vi "deleteDeviceLow.vi"(8 "error in (no error)":errorcluster, 9 "S/N IN":string, 10 "Device Type In":T1=enum."k4b2", 11 "reference in":refnum<class "Project Panels.lvclass">=refnum) -> (0 "error out":errorcluster={"status"=TRUE, "code"=1556, "source"="In Place Element Structure in File Controller.lvclass:getExcelFileRefs.vi->Devices Controller.lvclass:newDevice.vi->Project Panels.lvclass:newItem.vi->Project Panels.lvclass:products.vi->GUI Controller.lvclass:operate.vi->Master Controller.lvclass:operate.vi->main.vi"}, 2 "saved?":bool, 3 "reference out":refnum<class "Project Panels.lvclass">)   [LabVIEW 2016, in "Project Panels.lvclass"]
uses:
  Project Panels.lvclass
  SYS/Devices Controller_llb/deviceType.ctl
  deviceState.ctl
  SYS/Devices Controller_llb/Devices Controller.lvclass
panel:
  out "title":string="Deleting ...."
  out "O2 Exp Date (mm-aa)":string
  out "Serviced by":string
  out "O2 Last Changed (mm-aa)":string
  out "Follow Up Accepeted":string
  out "Follow Up Sent":string
  out "Device Type":T1=enum."k4b2"
  out "City":string
  out "End User Email":string
  out "End User":string
  out "System's Location":string
  out "Account":string
  out "Description":string
  out "SW Version":string
  out "S/N":string
  out "statusBar":string
  in  "Delete Item":bool
  in  "Stop Button":bool
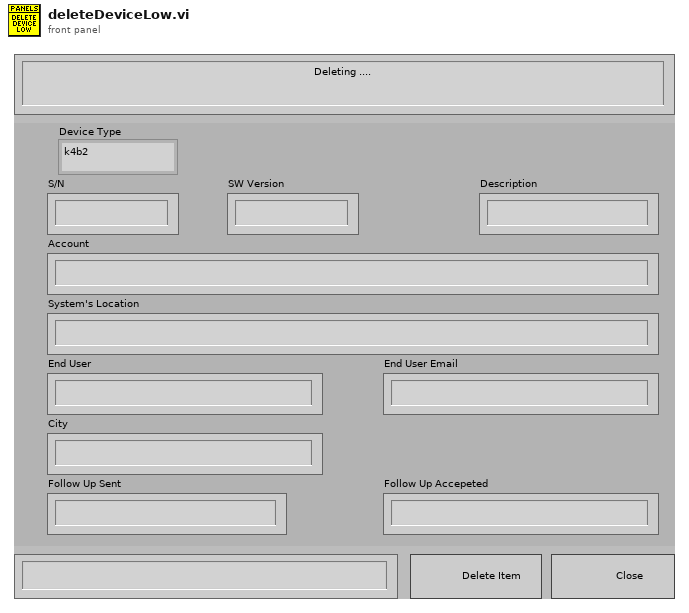
[diagram p1: front panel]
types:
  T1 = typedef "Devices Controller.lvclass/deviceType.ctl" = enum16{"k5", "k4b2", "fitmate", "cpet", "rmr", "bodyBoxPft", "bp", "pp"}
  T2 = cluster{"deviceType":T1, "S/N":string, "SW":string, "Description":string, "Account":string, "System's Location":string, "End User":string, "Email":string, "City":string, "LastChange":string, "Service By":string, "Exp Date":string, "FollowUp Sent":string, "FollowUp Accepted":string}
  T3 = typedef "Project Panels.lvclass/deviceState.ctl" = enum16{"check", "initiate", "waitEvent", "dataFromPDF", "getDetails", "TSR", "save", "close", "stop"}
  T4 = typedef "Project Panels.lvclass/ObjectAttributesRef.ctl" = refnum<data-value>
  T5 = typedef "Project Panels.lvclass/ObjectAttributes.ctl" = cluster{"MyAttribute":dbl, "device_controller_ref":refnum<class "Devices Controller.lvclass">, "file_controller_ref":refnum<class "File Controller.lvclass">, "item_controller_ref":refnum<class "Items Controller.lvclass">, "item_tables":cluster{"checkIN":string[][], "checkOUT":string[][], "storage":string[][]}, "quickbook_table":cluster{"notes":string[][]}, "notification_controller_ref":refnum<class "Notification Controller.lvclass">, "partstracking_controller_ref":refnum<class "PartsTracking Controller.lvclass">, "product_tables":cluster{"k4b2":string[][], "fitmate":string[][], "RMR":string[][], "CPET":string[][], "BP":string[][], "PP":string[][], "k5":string[][], "bb-pft":string[][]}, "rowsColour":u32[], "low_resolution?":bool, "run_python?":bool}
  T6 = cluster{"deviceType":T1, "S/N":string, "SW":string, "Description":string, "Account":string, "System's Location":string, "End User":string, "Email":string, "City":string, "LastChange":string, "Service By":string, "Exp Date":string, "FollowUp Sent":string, "FollowUp Accepted":string, "Note":string}
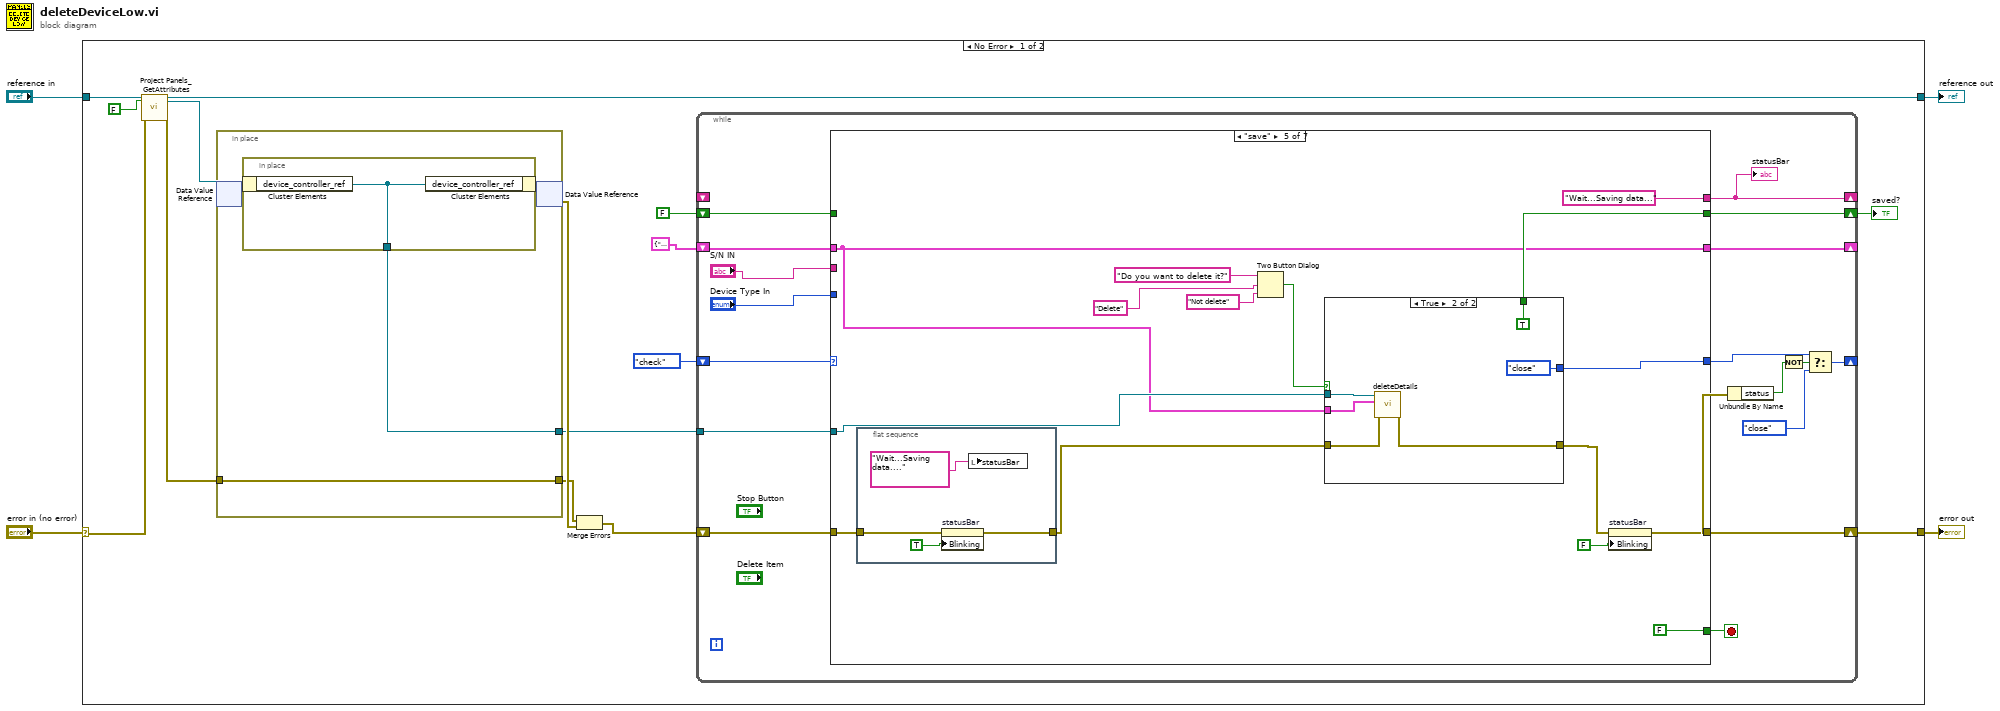
[diagram p0: block diagram]
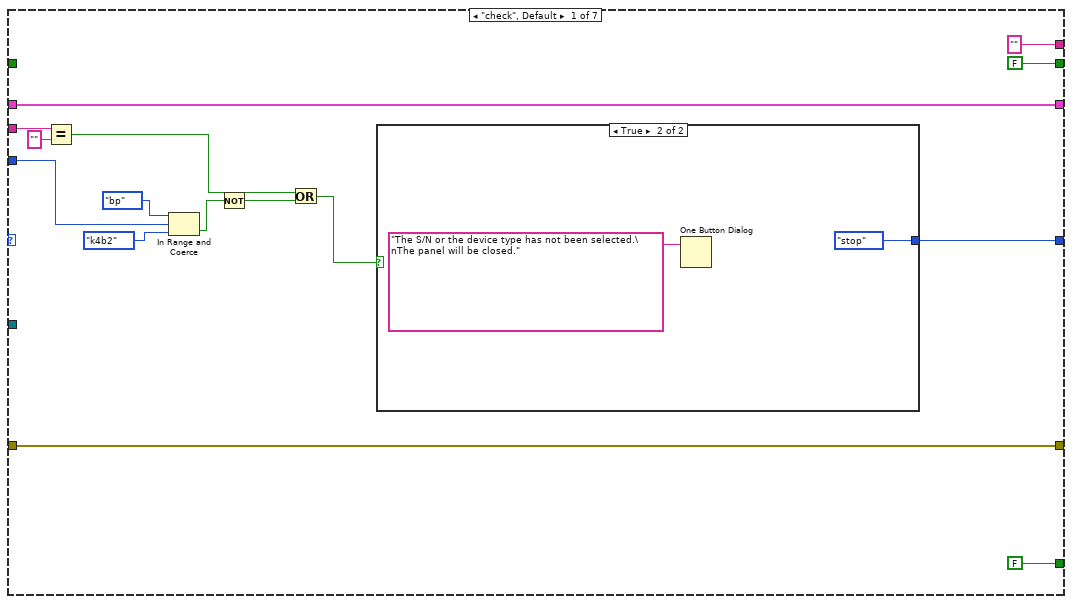
[diagram p2: hidden frame]
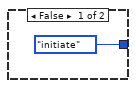
[diagram p3: hidden frame]
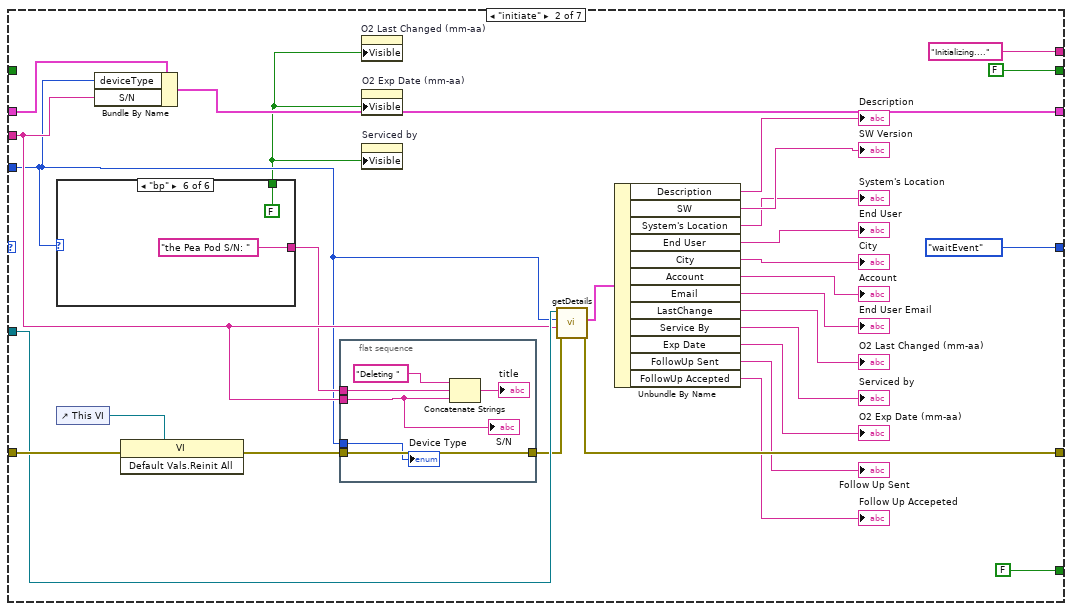
[diagram p4: hidden frame]
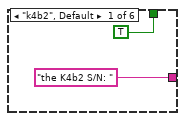
[diagram p5: hidden frame]
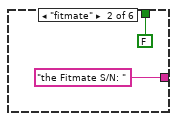
[diagram p6: hidden frame]
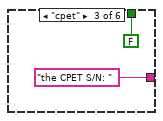
[diagram p7: hidden frame]
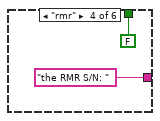
[diagram p8: hidden frame]
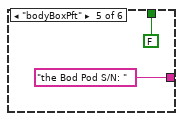
[diagram p9: hidden frame]
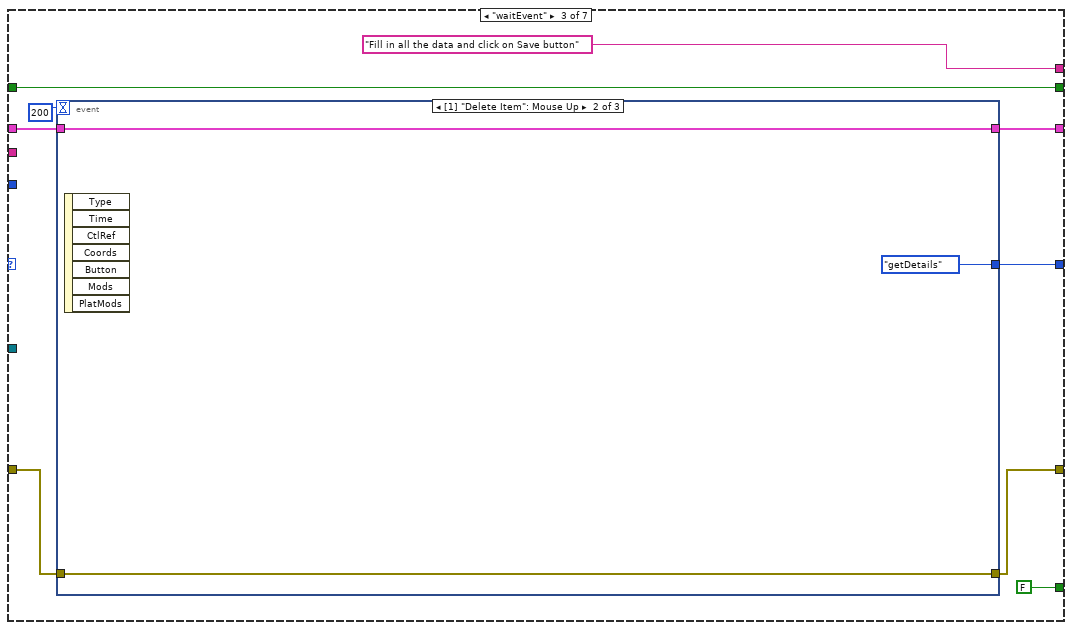
[diagram p10: hidden frame]
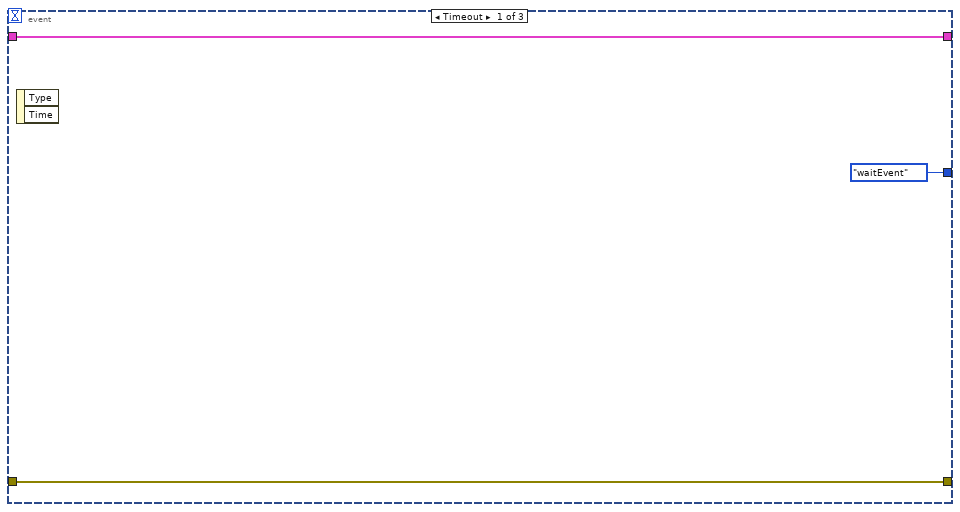
[diagram p11: hidden frame]
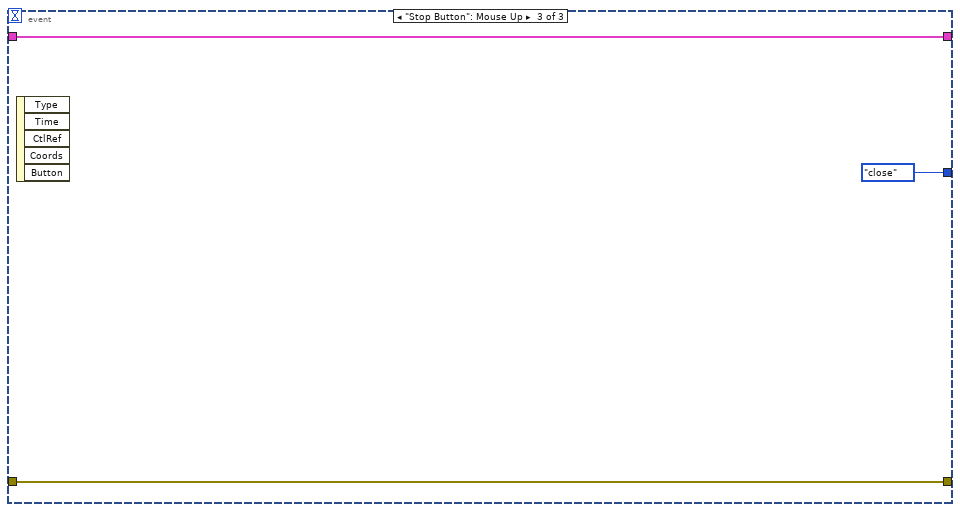
[diagram p12: hidden frame]
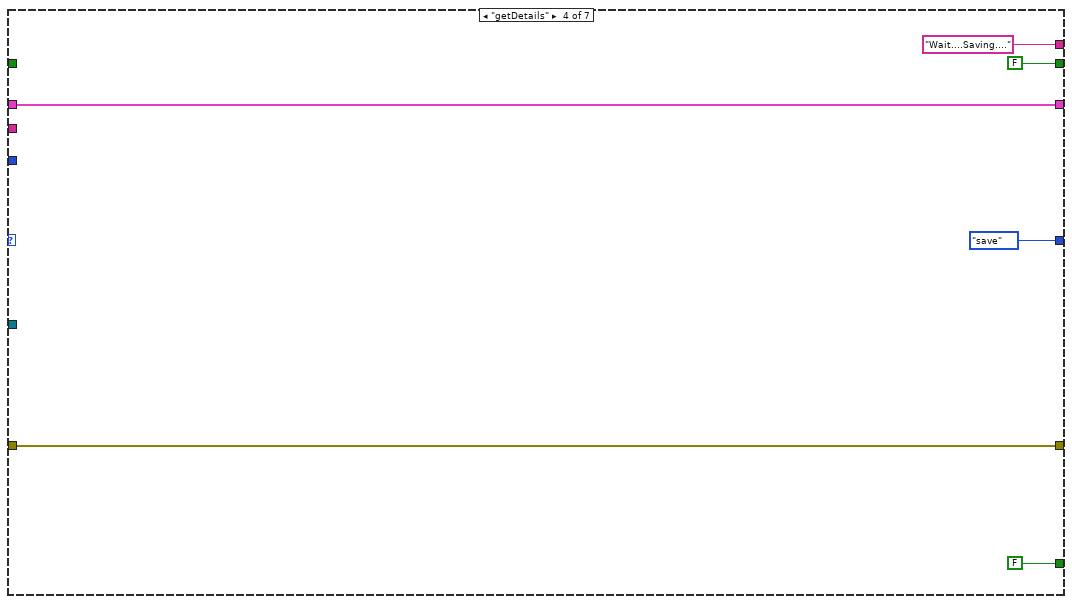
[diagram p13: hidden frame]
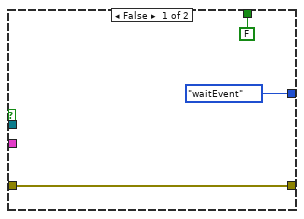
[diagram p14: hidden frame]
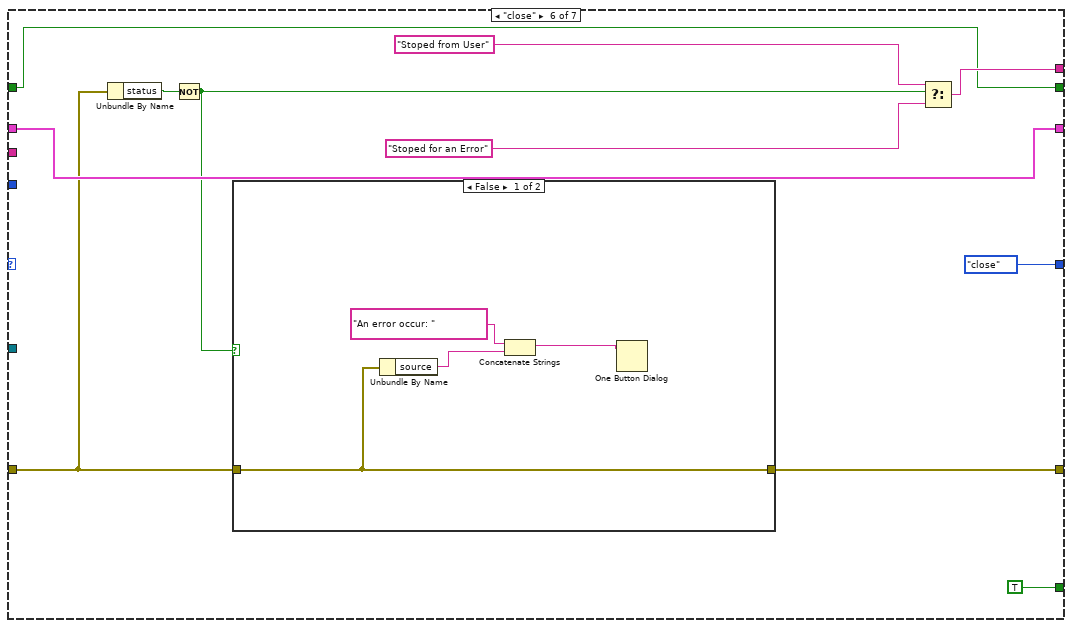
[diagram p15: hidden frame]
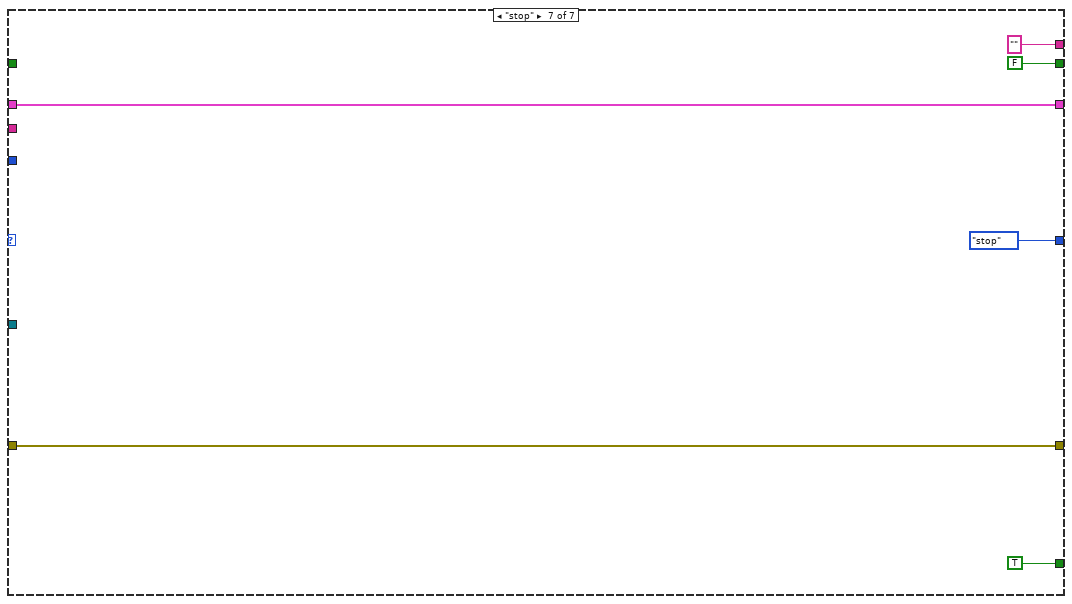
[diagram p17: hidden frame]
diagram:
  n1 = case shown="No Error" "error in (no error)" {
    selector: "error in (no error)" -> [w15 w182]
    tunnel: [w10 w182] -> w3
    tunnel: [w13 w181] -> w1
    tunnel: "reference in" -> [w17 w181]
    frame No Error {
      n2 = call "Project Panels_GetAttributes.vi"("reference in"=w17, "return data? (T)"=FALSE, "error in (no error)"=w15) -> ("reference out"=w13:refnum<class "Project Panels.lvclass">, "attributes ref"=w12:T4, "error out"=w14:errorcluster)  [unwired: 13 in, 1 out]
      n3 = in-place {
        in-place-border: w14 -> [w177]
        in-place-border: [w177] -> w18
        in-place-border: [w176] -> w8
        n4 = in-place-dvr #1(w12) -> (w178:T5)  [unwired: 1 out]
        n5 = in-place {
          in-place-border: [w180] -> w176
          n6 = in-place-cluster #2(w178) -> ("device_controller_ref"=w180:refnum<class "Devices Controller.lvclass">)
          n7 = in-place-cluster #2("device_controller_ref"=w180) -> (w179:T5)
        }
        n8 = in-place-dvr #1(w179) -> (w19:errorcluster)  [unwired: 1 out]
      }
      n9 = Merge Errors(w18, w19) -> (w11:errorcluster)
      n10 = while {
        shift-right: [w25] -> w10
        shift-left: w11 -> [w36]
        shift-right: [w26] -> _
        shift-left: deviceState."check" ("state") -> [w35]
        shift-right: [w33] -> _
        shift-left: T2 {"deviceType"=enum."k5", "S/N"="", "SW"="", "Description"="", "Account"="", "System's Location"="", "End User"="", "Email"="", "City"="", "LastChange"="", "Service By"="", "Exp Date"="", "FollowUp Sent"="", "FollowUp Accepted"=""} ("details") -> [w32]
        shift-right: [w31] -> _
        shift-left: _ -> [_]
        tunnel: w8 -> [w30]
        shift-right: [w29] -> w5
        shift-left: FALSE -> [w28]
        stop <- w34 stop-if-true
        n11 = case shown="\"save\"" w35 {
          tunnel: w36 -> [w51 w78 w105 w125 w135 w159 w174]
          tunnel: [w51 w77 w104 w125 w132 w158 w174] -> w25
          tunnel: [FALSE FALSE FALSE FALSE FALSE TRUE TRUE] -> w34
          tunnel: [w38 deviceState."waitEvent" ("state") w109 deviceState."save" ("f") w139 deviceState."close" ("f") deviceState."stop" ("f")] -> w27
          tunnel: "Device Type In" -> [w47 w68 _ _ _ _ _]
          tunnel: [w48 w73 w102 w120 w136 w161 w172] -> w33
          tunnel: w32 -> [w48 w74 w103 w120 w136 w161 w172]
          tunnel: ["" ("title") "Initializing...." ("statusBar") "Fill in all the data and click on Save button" ("statusBar") "Wait....Saving...." ("title") "Wait...Saving data..." ("title") w160 "" ("title")] -> w31
          tunnel: w30 -> [_ w76 _ _ w138 _ _]
          tunnel: [FALSE FALSE w106 FALSE w137 w156 FALSE] -> w29
          tunnel: w28 -> [_ _ w106 _ _ w156 _]
          tunnel: "S/N IN" -> [w44 w72 _ _ _ _ _]
          frame "check", Default {
            n12 = Equal?(x=w44, y="") -> (x = y?=w41:bool)
            n13 = In Range and Coerce(upper limit=deviceType."bp", x=w47, lower limit=deviceType."k4b2") -> (In Range?=w42:bool)  [unwired: 1 out]
            n14 = Not(x=w42) -> (.not. x?=w40:bool)
            n15 = Or(x=w41, y=w40) -> (x .or. y?=w39:bool)
            n16 = case shown="True" w39 {
              tunnel: [deviceState."initiate" ("f") deviceState."stop" ("f")] -> w38
              frame False {
              }
              frame True {
                n17 = One Button Dialog(message="The S/N or the device type has not been selected.\nThe panel will be closed.") -> ()  [unwired: 1 in, 1 out]
              }
            }
          }
          frame "initiate" {
            n18 = case shown="\"bp\"" w68 {
              tunnel: ["the K4b2 S/N: " ("string") "the Fitmate S/N: " ("string") "the CPET S/N: " ("string") "the RMR S/N: " ("string") "the Bod Pod S/N: " ("string") "the Pea Pod S/N: " ("string")] -> w71
              tunnel: [TRUE ("Visible") FALSE ("Visible") FALSE ("Visible") FALSE ("Visible") FALSE ("Visible") FALSE ("Visible")] -> w67
              frame "k4b2", Default {
              }
              frame "fitmate" {
              }
              frame "cpet" {
              }
              frame "rmr" {
              }
              frame "bodyBoxPft" {
              }
              frame "bp" {
              }
            }
            n19 = control-ref of="This VI"() -> (w79:refnum<vi>)
            n20 = Bundle By Name(cluster=w74, "deviceType"=w68, "S/N"=w72) -> (w73:T2)
            n21 = invoke class="VI" method="Default Vals.Reinit All"(reference=w79, error in=w78) -> (error out=w70:errorcluster)  [unwired: 1 in, 2 out]
            n22 = flat-sequence {
              tunnel: w72 -> [w85]
              tunnel: w71 -> [w87]
              tunnel: w70 -> [w86]
              tunnel: [w86] -> w69
              tunnel: w68 -> [w84]
              frame #0 {
                n23 = Concatenate Strings("Deleting " ("title"), w87, w85) -> (→"title":string)
                "S/N" <- w85
                "Device Type" <- w84
              }
            }
            n24 = property on="O2 Last Changed (mm-aa)" class="Str"("Visible"=w67) -> ()  [unwired: 2 in, 2 out]
            n25 = property on="O2 Exp Date (mm-aa)" class="Str"("Visible"=w67) -> ()  [unwired: 2 in, 2 out]
            n26 = property on="Serviced by" class="Str"("Visible"=w67) -> ()  [unwired: 2 in, 2 out]
            n27 = call "getDetails.vi"("error in (no error)"=w69, "S/N"=w72, "Device Type"=w68, "reference in"=w76) -> ("error out"=w77:errorcluster, "details"=w75:T6)  [unwired: 5 in, 1 out]
            n28 = Unbundle By Name(w75) -> ("Description"=→"Description":string, "SW"=→"SW Version":string, "System's Location"=→"System's Location":string, "End User"=→"End User":string, "City"=→"City":string, "Account"=→"Account":string, "Email"=→"End User Email":string, "LastChange"=→"O2 Last Changed (mm-aa)":string, "Service By"=→"Serviced by":string, "Exp Date"=→"O2 Exp Date (mm-aa)":string, "FollowUp Sent"=→"Follow Up Sent":string, "FollowUp Accepted"=→"Follow Up Accepeted":string)
          }
          frame "waitEvent" {
            n29 = event shown="[1] \"Delete Item\": Mouse Up" {
              selector: _ -> [_ _ _]
              dyn-events: _ -> [_ _ _]
              timeout: 200 -> [_ _ _]
              tunnel: [deviceState."waitEvent" ("state") deviceState."getDetails" ("state") deviceState."close" ("state")] -> w109
              tunnel: [w112 w115 w118] -> w104
              tunnel: w105 -> [w112 w115 w118]
              tunnel: w103 -> [w111 w114 w117]
              tunnel: [w111 w114 w117] -> w102
              event Timeout {
                n30 = event-data() -> ()  [unwired: 1 in, 2 out]
              }
              event "Delete Item": Mouse Up {
                n31 = event-data() -> ()  [unwired: 1 in, 7 out]
              }
              event "Stop Button": Mouse Up {
                n32 = event-data() -> ()  [unwired: 1 in, 5 out]
              }
            }
          }
          frame "getDetails" {
          }
          frame "save" {
            n33 = flat-sequence {
              tunnel: [w151] -> w134
              tunnel: w135 -> [w152]
              frame #0 {
                n34 = property on="statusBar" class="Str"(error in=w152, "Blinking"=TRUE) -> (error out=w151:errorcluster)  [unwired: 1 in, 1 out]
                n35 = local write "statusBar"("Wait...Saving data...." ("statusBar")) -> ()
              }
            }
            n36 = Two Button Dialog(message="Do you want to delete it?", 1:"Not delete" ("F button name (\"Cancel\")"), 2:"Delete" ("T button name (\"OK\")")) -> (T button?=w128:bool)
            n37 = case shown="True" w128 {
              tunnel: [deviceState."waitEvent" ("state") deviceState."close" ("state")] -> w139
              tunnel: w134 -> [w143 w148]
              tunnel: w138 -> [_ w147]
              tunnel: w136 -> [_ w146]
              tunnel: [w143 w144] -> w131
              tunnel: [FALSE TRUE] -> w137
              frame False {
              }
              frame True {
                n38 = call "deleteDetails.vi"("error in (no error)"=w148, "details"=w146, "reference in"=w147) -> ("error out"=w144:errorcluster)  [unwired: 7 in, 1 out]
              }
            }
            n39 = property on="statusBar" class="Str"(error in=w131, "Blinking"=FALSE) -> (error out=w132:errorcluster)  [unwired: 1 in, 1 out]
          }
          frame "close" {
            n40 = Unbundle By Name(w159) -> ("status"=w164:bool)
            n41 = Not(x=w164) -> (.not. x?=w157:bool)
            n42 = case shown="False" w157 {
              tunnel: w159 -> [w166 w169]
              tunnel: [w166 w169] -> w158
              frame False {
                n43 = Unbundle By Name(w166) -> ("source"=w165:string)
                n44 = Concatenate Strings("An error occur: " ("message"), w165) -> (w167:string)
                n45 = One Button Dialog(message=w167) -> ()  [unwired: 1 in, 1 out]
              }
              frame True {
              }
            }
            n46 = Select(t="Stoped from User" ("title"), s=w157, f="Stoped for an Error" ("title")) -> (s? t:f=w160:string)
          }
          frame "stop" {
          }
        }
        "statusBar" <- w31
        n47 = Unbundle By Name(w25) -> ("status"=w24:bool)
        n48 = Not(x=w24) -> (.not. x?=w22:bool)
        n49 = Select(t=w27, s=w22, f=deviceState."close") -> (s? t:f=w26:T3)
      }
      "saved?" <- w5
    }
    frame Error {
    }
  }
  "error out" <- w3
  "reference out" <- w1
